vi "Moonlanding.vi"() -> ()   [LabVIEW 2012]
doc: "This example is a game that shows the power of the Express VIs. \n\nLanding on the Moon: Drop from 10000 meters and land at 5 m/s or less .\n\nThis example uses the following Express VIs: Formula, Trigger and Gate, Comparison, and Display Message to User."
uses:
  Instance           5 19Saved   Moonlanding .vi
  Instance           3 19Saved   Moonlanding .vi
  Instance           4 19Saved   Moonlanding .vi
  Instance           1 19Saved   Moonlanding .vi
  Instance           2 19Saved   Moonlanding .vi
  <vilib>/express/express shared/transition.llb/Dynamic To Waveform Array.vi
  <vilib>/express/express shared/transition.llb/Waveform Array To Dynamic.vi
  <vilib>/express/express arith-compare/Formula/Block/exnFormulaBlock how many pts in the wave.vi
  <vilib>/express/express shared/ex_Modify Signal Name.vi
  <vilib>/express/express arith-compare/Formula/XNode/ExpressFormulaBlockNode.xnode
panel:
  in  "Message":string="You Win!"
  out "Speed":dbl(knob) scale=-200.0..200.0
  out "Fuel":dbl format="%0.2f"
  out "Speed":dbl format="%0.2f"
  out "Altitude Chart":dynamicdata(graph)
  out "Speed":dbl(knob) scale=-30.0..30.0
  out "Height":dbl(knob) scale=0.0..1000.0
  out "Height":dbl(knob) scale=0.0..10000.0
  out "Tank":dbl(slide) scale=0.0..50000.0
  in  "Power":dbl(slide) scale=0.0..100.0
  # "Landing on the Moon\nDrop from 10000 meters and land at 5 m/s or less."
  # "Normal Flight"
  # "Final Approach"
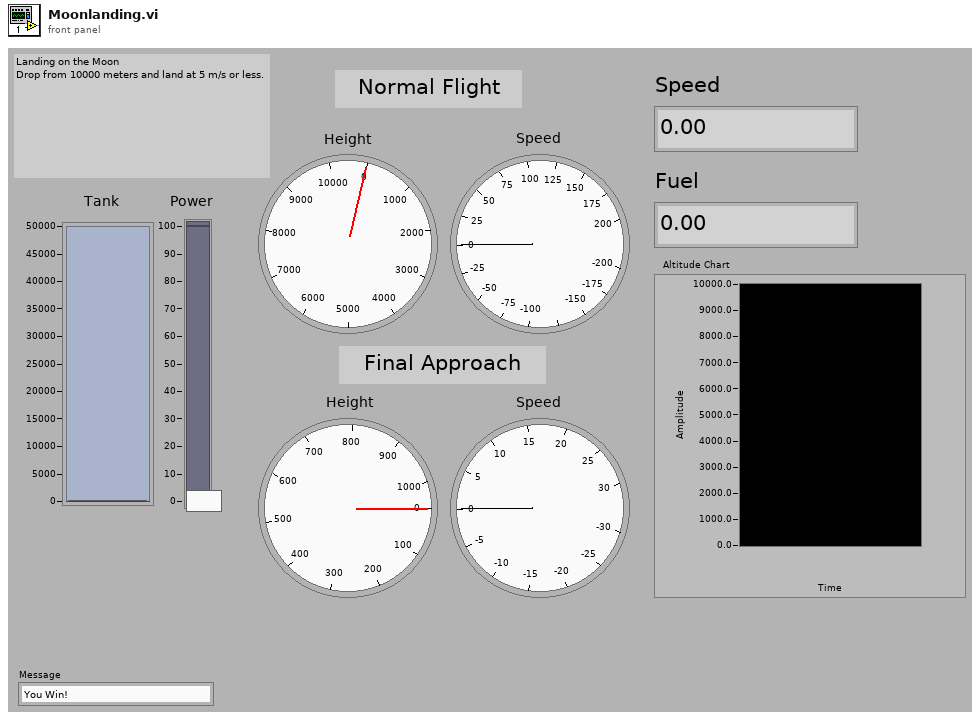
[diagram p1: front panel]
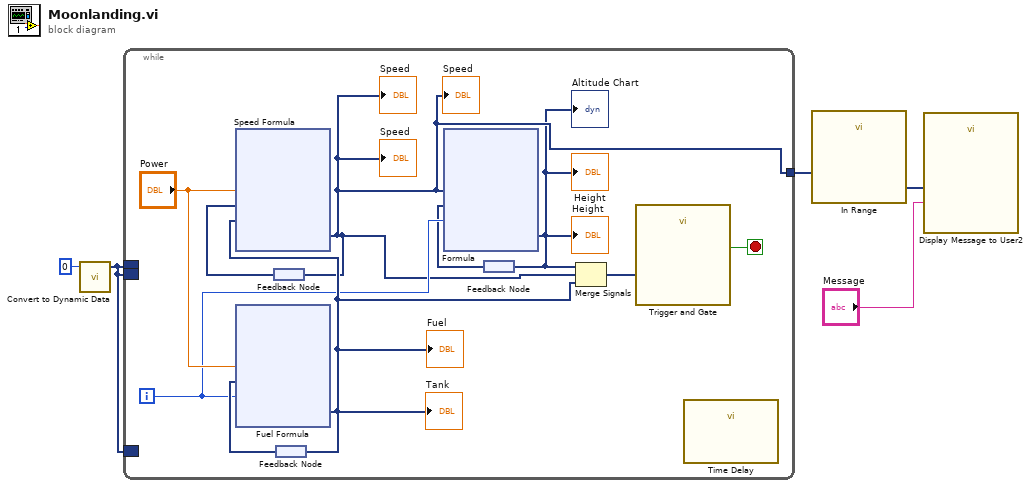
[diagram p0: block diagram]
diagram:
  n1 = call "Convert to Dynamic Data"("Double"=0) -> ("Dynamic Data Type"=w4:dynamicdata)  [unwired: 3 out]
  n2 = while {
    tunnel: [w8] -> w3
    border: w4 -> [_]
    border: w4 -> [_]
    border: w4 -> [_]
    i -> [w9]
    stop <- w15 stop-if-true
    n3 = feedback #1() -> (w13:dynamicdata)
    n4 = feedback #2() -> (w11:dynamicdata)
    n5 = xnode "Fuel Formula"("Power"="Power", "LastFuel"=w11, "Iteration"=w9) -> ("Result"=w10:dynamicdata)  [unwired: 1 in, 1 out]
    "Tank" <- w10
    "Fuel" <- w10
    n6 = xnode "Speed Formula"("Power"="Power", "LastSpeed"=w13, "Fuel"=w10) -> ("Result"=w8:dynamicdata)  [unwired: 1 in, 1 out]
    "Speed" <- w8
    "Speed" <- w8
    "Speed" <- w8
    n7 = feedback-in #1(w8) -> ()
    n8 = feedback-in #2(w10) -> ()
    n9 = feedback #3() -> (w7:dynamicdata)
    n10 = xnode "Formula"("Speed"=w8, "LastHeight"=w7, "Iteration"=w9) -> ("Result"=w6:dynamicdata)  [unwired: 1 in, 1 out]
    "Height" <- w6
    "Height" <- w6
    "Altitude Chart" <- w6
    n11 = feedback-in #3(w6) -> ()
    n12 = Merge Signals(w6, w8, w10) -> (w14:dynamicdata)
    n13 = call "Trigger and Gate"("Signals"=w14) -> ("Data Available"=w15:bool)  [unwired: 4 in, 6 out]
    n14 = call "Time Delay"() -> ()  [unwired: 2 in, 10 out]
  }
  n15 = call "In Range"("Operand 1"=w3) -> ("Result"=w2:dynamicdata)  [unwired: 1 in, 9 out]
  n16 = call "Display Message to User2"("Enable"=w2, "Message"="Message") -> ()  [unwired: 1 in, 9 out]
